vi "test Get and Set Debug Flags.vi"(8 "error in (no error)":errorcluster, 11 "TestCase in":refnum<class "Framework Property Tests.lvclass">) -> (0 "error out":errorcluster, 3 "TestCase out":refnum<class "Framework Property Tests.lvclass">)   [LabVIEW 2017, in "Framework Property Tests.lvclass"]
uses:
  Framework Property Tests.lvclass
  <vilib>/addons/_JKI Toolkits/VI Tester/TestCase.llb/TestCase.lvclass
  Engine/Classes/Debug/Debug Flags/Debug Flags.lvclass
  Engine/Classes/Debug/FIFO Flags/FIFO Flags.lvclass
  Classes/Framework/Framework.lvclass
  C:/Program Files (x86)/National Instruments/LabVIEW 2017/vi.lib/addons/_JKI Toolkits/VI Tester/TestCase.llb/TestCase.lvclass
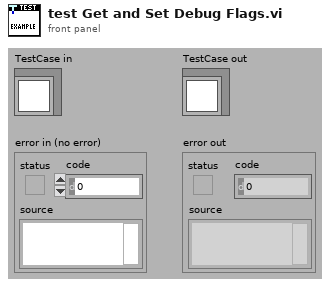
[diagram p1: front panel]
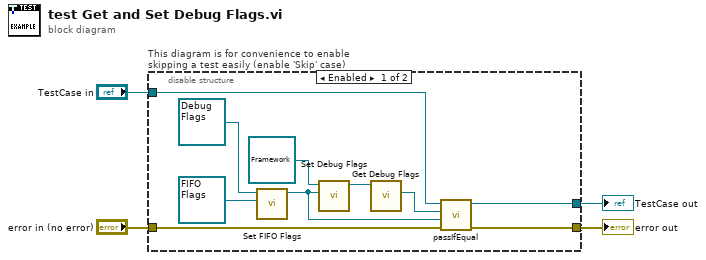
[diagram p0: block diagram]
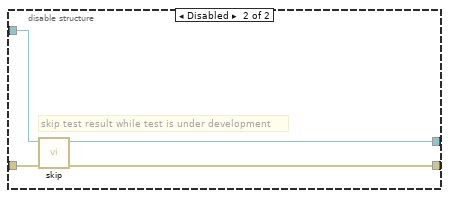
[diagram p2: hidden frame]
diagram:
  n1 = disable-structure "This diagram is for convenience to enable skipping a test easily (enable 'Skip' case)" shown="Enabled" {
    disable-tunnel: "TestCase in" -> [w12 w18]
    disable-tunnel: [w11 w16] -> w2
    disable-tunnel: [w13 w17] -> w1
    disable-tunnel: "error in (no error)" -> [w14 w15]
    frame Enabled {
      n2 = call "Set FIFO Flags.vi"("FIFO"=refnum<class "FIFO Flags.lvclass"> refnum, "Debug Flags in"=refnum<class "Debug Flags.lvclass"> refnum ("DSF Core.lvlib:Debug Flags.lvclass")) -> ("Debug Flags out"=w6:refnum<class "Debug Flags.lvclass">)  [unwired: 9 in]
      n3 = call "Set Debug Flags.vi"("Debug Flags"=w6, "Framework in"=refnum<class "Framework.lvclass"> refnum ("Mock Framework in")) -> ("Framework out"=w8:refnum<class "Framework.lvclass">)  [unwired: 9 in]
      n4 = call "Get Debug Flags.vi"("Framework in"=w8) -> ("Debug Flags"=w7:refnum<class "Debug Flags.lvclass">)  [unwired: 9 in, 1 out]
      n5 = call-dynamic "passIfEqual.vi"("error in (no error)"=w14, "y"=w6, "x"=w7, "TestCase in"=w12) -> ("error out"=w13:errorcluster, "TestCase out"=w11:refnum<class "Framework Property Tests.lvclass">)  [unwired: 6 in]
    }
    frame Disabled {
      # "skip test result while test is under development"
      n6 = call <vilib>:"skip.vi"("error in (no error)"=w15, "TestCase in"=w18) -> ("error out"=w17:errorcluster, "TestCase out"=w16:refnum<class "Framework Property Tests.lvclass">)  [unwired: 8 in]
    }
  }
  "error out" <- w1
  "TestCase out" <- w2
